vi "source_check_compliance_from_device.vi"(8 "error in (no error)":errorcluster, 11 "VISA resource name":refnum<visa-resource-name>) -> (0 "error out":errorcluster, 2 "Value":sgl, 3 "VISA resource name out":refnum<visa-resource-name>)   [LabVIEW 2016]
panel:
  out "return count":u32
  out "read buffer":string
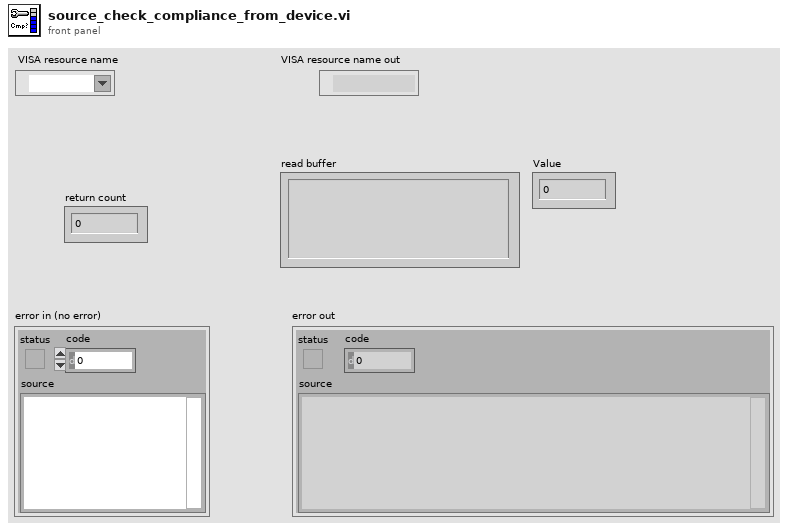
[diagram p1: front panel]
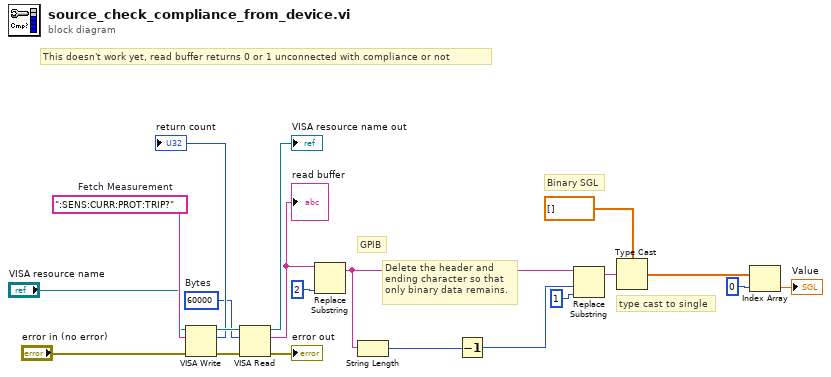
[diagram p0: block diagram]
diagram:
  w20 = ":SENS:CURR:PROT:TRIP?"  # Fetch Measurement
  w14 = u32 60000  # Bytes
  # "This doesn't work yet, read buffer returns 0 or 1 unconnected with compliance or not"
  # "Binary SGL"
  # "Delete the header and ending character so that only binary data remains."
  # "GPIB"
  # "type cast to single"
  n1 = VISA Write(VISA resource name="VISA resource name", write buffer=w20, error in (no error)="error in (no error)") -> (VISA resource name out=w17:refnum<visa-resource-name>, return count=→"return count":u32, error out=w16:errorcluster)
  n2 = VISA Read(VISA resource name=w17, byte count=w14, error in (no error)=w16) -> (VISA resource name out=→"VISA resource name out":refnum<visa-resource-name>, read buffer=w4:string, error out=→"error out":errorcluster)  [unwired: 1 out]
  "read buffer" <- w4
  n3 = Replace Substring(2:2 ("length (len. of substring)"), 5:w4) -> (1:w12:string)  [unwired: 2 in, 1 out]
  n4 = String Length(string=w12) -> (length=w11:i32)
  n5 = Decrement(x=w11) -> (x-1=w10:i32)
  n6 = Replace Substring(2:1 ("length (len. of substring)"), 3:w10, 5:w12) -> (1:w7:string)  [unwired: 1 in, 1 out]
  n7 = Type Cast(type=sgl[] [], x=w7) -> (*(type *) &x=w6:sgl[])
  n8 = Index Array(array=w6, index=0) -> (element=→"Value":sgl)
